vi "Robot_s First Move.vi"(0 "VISA Refnum in":refnum<visa-resource-name>="ASRL5::INSTR", 5 "In Play Array":i32[](array[numeric])=[-1, -1, -1, -1, -1, -1, -1, -1, -1, -1, -1, -1, -1, -1, -1, -1, -1, -1], 9 "Current Image Array 2":i32[](array[numeric])=[-1, -1, -1, -1, -1, -1, -1, -1, -1, -1, -1, -1, -1, -1, -1, -1, -1, -1]) -> (4 "VISA Refnum out":refnum<visa-resource-name>="ASRL5::INSTR", 6 "Index From First Move":i32=17, 8 "Image Value from First Turn":i32=4, 10 "Output Image Array":i32[](array[numeric]), 15 "error out":errorcluster={"status"=FALSE, "code"=1073676294, "source"="VISA Read in Read from Machine.vi->ReadUarmCoordinatesCompareV3.vi->Move_Until_Home.vi->RobotTurnMovement.vi->Robot_s First Move.vi"})   [LabVIEW 2018]
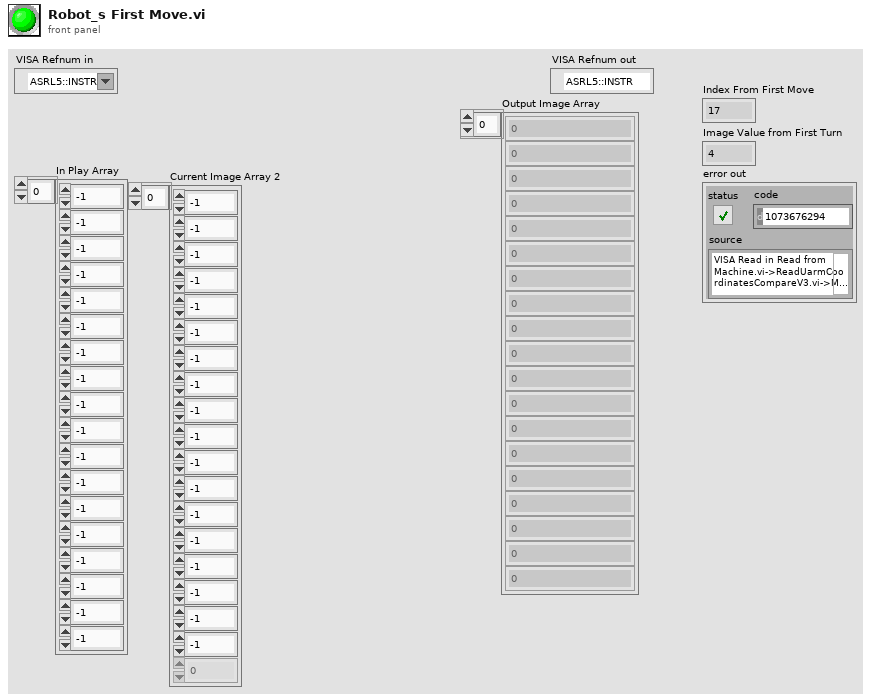
[diagram p1: front panel]
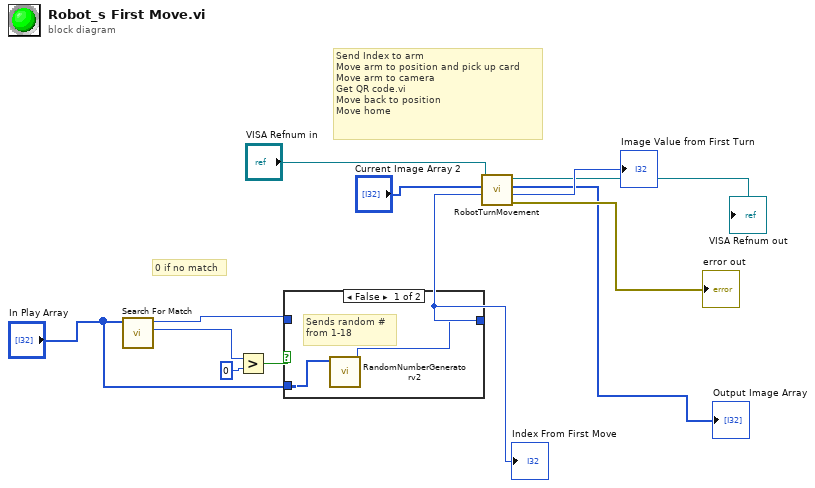
[diagram p0: block diagram]
diagram:
  # "0 if no match"
  # "Send Index to arm\nMove arm to position and pick up card\nMove arm to camera\nGet QR code.vi\nMove back to position\nMove home"
  n1 = call "Search For Match.vi"("Array"="In Play Array") -> ("Index 2"=w12:i32, "Index 1"=w10:i32)  [unwired: 9 in]
  n2 = Greater?(x=w12, y=0) -> (0:w9:bool)
  n3 = case shown="False" w9 {
    tunnel: w10 -> [_ w15]
    tunnel: [w14 w15] -> w6
    tunnel: "In Play Array" -> [w13 _]
    frame False {
      # "Sends random # \nfrom 1-18"
      n4 = call "RandomNumberGeneratorv2.vi"("In Play Array"=w13) -> ("Index"=w14:u8)  [unwired: 10 in]
    }
    frame True {
    }
  }
  "Index From First Move" <- w6
  n5 = call "RobotTurnMovement.vi"("index"=w6, "Current Image Array"="Current Image Array 2", "VISA Refnum in"="VISA Refnum in") -> ("error out"=→"error out":errorcluster, "Image Value"=→"Image Value from First Turn":i32, "Output Array"=→"Output Image Array":i32[], "VISA Refnum out"=→"VISA Refnum out":refnum<visa-resource-name>)  [unwired: 5 in]
